vi "sensor integration for debug async v5.vi"() -> ()   [LabVIEW 2021]
uses:
  <vilib>/Analysis/NI_AALBase.lvlib
  65c7c016-c5e7-4ca0-8b30-908e1d77d521.vi
  <vilib>/Instr/_visa.llb/VISA Configure Serial Port (Instr).vi
  <vilib>/Analysis/baseanly.llb/Mean (DBL).vi
  controls/sensirion_flow_sensor_data.ctl
  type-defs/sensirion_data_with_time.ctl
  <extravilib>/ChannelInstances/Stream-t'sensirion_data_with_time.ctl'.lvlib
panel:
  out "sensor data timestamp":dbl
  out "logfile size (in MB)":dbl format="%.2f"
  out "sensirion data string":string
  in  "error in (no error)":errorcluster
  out "retry count":i32
  in  "read byte count (512)":u32=512
  in  "baud rate (576000)":u32=576000
  out "last loop time, ms":dbl
  out "mean refresh rate, Hz, n=250":dbl(knob) scale=0.05..100.0
  in  "loop delay, ms (0)":u32
  in  "expected num sensors (12)":i32=12
  out "sensor data array 7 - 12":T1[](array[typedef])=[{"flow rate \n(mL/min)"=0.0, "flow val. status"=FALSE, "temp.\n(C)"=0.0, "temp. val status"=FALSE, "air in \nline?"=FALSE, "high \nflow?"=FALSE, "flag. val status"=FALSE}, {"flow rate \n(mL/min)"=0.0, "flow val. status"=FALSE, "temp.\n(C)"=0.0, "temp. val status"=FALSE, "air in \nline?"=FALSE, "high \nflow?"=FALSE, "flag. val status"=FALSE}, {"flow rate \n(mL/min)"=0.0, "flow val. status"=TRUE, "temp.\n(C)"=0.0, "temp. val status"=TRUE, "air in \nline?"=FALSE, "high \nflow?"=FALSE, "flag. val status"=TRUE}, {"flow rate \n(mL/min)"=0.0, "flow val. status"=TRUE, "temp.\n(C)"=0.0, "temp. val status"=TRUE, "air in \nline?"=FALSE, "high \nflow?"=FALSE, "flag. val status"=TRUE}, {"flow rate \n(mL/min)"=0.0, "flow val. status"=TRUE, "temp.\n(C)"=0.0, "temp. val status"=TRUE, "air in \nline?"=FALSE, "high \nflow?"=FALSE, "flag. val status"=TRUE}, {"flow rate \n(mL/min)"=0.0, "flow val. status"=TRUE, "temp.\n(C)"=0.0, "temp. val status"=TRUE, "air in \nline?"=FALSE, "high \nflow?"=FALSE, "flag. val status"=TRUE}, {"flow rate \n(mL/min)"=0.0, "flow val. status"=TRUE, "temp.\n(C)"=0.0, "temp. val status"=TRUE, "air in \nline?"=FALSE, "high \nflow?"=FALSE, "flag. val status"=TRUE}, {"flow rate \n(mL/min)"=0.0, "flow val. status"=TRUE, "temp.\n(C)"=0.0, "temp. val status"=TRUE, "air in \nline?"=FALSE, "high \nflow?"=FALSE, "flag. val status"=TRUE}, {"flow rate \n(mL/min)"=0.0, "flow val. status"=TRUE, "temp.\n(C)"=0.0, "temp. val status"=TRUE, "air in \nline?"=FALSE, "high \nflow?"=FALSE, "flag. val status"=TRUE}, {"flow rate \n(mL/min)"=0.0, "flow val. status"=TRUE, "temp.\n(C)"=0.0, "temp. val status"=TRUE, "air in \nline?"=FALSE, "high \nflow?"=FALSE, "flag. val status"=TRUE}, {"flow rate \n(mL/min)"=0.0, "flow val. status"=TRUE, "temp.\n(C)"=0.0, "temp. val status"=TRUE, "air in \nline?"=FALSE, "high \nflow?"=FALSE, "flag. val status"=TRUE}, {"flow rate \n(mL/min)"=0.0, "flow val. status"=TRUE, "temp.\n(C)"=0.0, "temp. val status"=TRUE, "air in \nline?"=FALSE, "high \nflow?"=FALSE, "flag. val status"=TRUE}] {"temp.\n(C)" scale=20.0..30.0 scale format="%#_3g"; "flow rate \n(mL/min)" scale=0.0..4.0}
  out "sensor data array 1 - 6":T1[](array[typedef])=[{"flow rate \n(mL/min)"=0.0, "flow val. status"=FALSE, "temp.\n(C)"=0.0, "temp. val status"=FALSE, "air in \nline?"=FALSE, "high \nflow?"=FALSE, "flag. val status"=FALSE}, {"flow rate \n(mL/min)"=0.0, "flow val. status"=FALSE, "temp.\n(C)"=0.0, "temp. val status"=FALSE, "air in \nline?"=FALSE, "high \nflow?"=FALSE, "flag. val status"=FALSE}, {"flow rate \n(mL/min)"=0.0, "flow val. status"=TRUE, "temp.\n(C)"=0.0, "temp. val status"=TRUE, "air in \nline?"=FALSE, "high \nflow?"=FALSE, "flag. val status"=TRUE}, {"flow rate \n(mL/min)"=0.0, "flow val. status"=TRUE, "temp.\n(C)"=0.0, "temp. val status"=TRUE, "air in \nline?"=FALSE, "high \nflow?"=FALSE, "flag. val status"=TRUE}, {"flow rate \n(mL/min)"=0.0, "flow val. status"=TRUE, "temp.\n(C)"=0.0, "temp. val status"=TRUE, "air in \nline?"=FALSE, "high \nflow?"=FALSE, "flag. val status"=TRUE}, {"flow rate \n(mL/min)"=0.0, "flow val. status"=TRUE, "temp.\n(C)"=0.0, "temp. val status"=TRUE, "air in \nline?"=FALSE, "high \nflow?"=FALSE, "flag. val status"=TRUE}, {"flow rate \n(mL/min)"=0.0, "flow val. status"=TRUE, "temp.\n(C)"=0.0, "temp. val status"=TRUE, "air in \nline?"=FALSE, "high \nflow?"=FALSE, "flag. val status"=TRUE}, {"flow rate \n(mL/min)"=0.0, "flow val. status"=TRUE, "temp.\n(C)"=0.0, "temp. val status"=TRUE, "air in \nline?"=FALSE, "high \nflow?"=FALSE, "flag. val status"=TRUE}, {"flow rate \n(mL/min)"=0.0, "flow val. status"=TRUE, "temp.\n(C)"=0.0, "temp. val status"=TRUE, "air in \nline?"=FALSE, "high \nflow?"=FALSE, "flag. val status"=TRUE}, {"flow rate \n(mL/min)"=0.0, "flow val. status"=TRUE, "temp.\n(C)"=0.0, "temp. val status"=TRUE, "air in \nline?"=FALSE, "high \nflow?"=FALSE, "flag. val status"=TRUE}, {"flow rate \n(mL/min)"=0.0, "flow val. status"=TRUE, "temp.\n(C)"=0.0, "temp. val status"=TRUE, "air in \nline?"=FALSE, "high \nflow?"=FALSE, "flag. val status"=TRUE}, {"flow rate \n(mL/min)"=0.0, "flow val. status"=TRUE, "temp.\n(C)"=0.0, "temp. val status"=TRUE, "air in \nline?"=FALSE, "high \nflow?"=FALSE, "flag. val status"=TRUE}] {"temp.\n(C)" scale=20.0..30.0 scale format="%#_3g"; "flow rate \n(mL/min)" scale=0.0..3.0}
  out "error out":errorcluster
  in  "stop program":bool
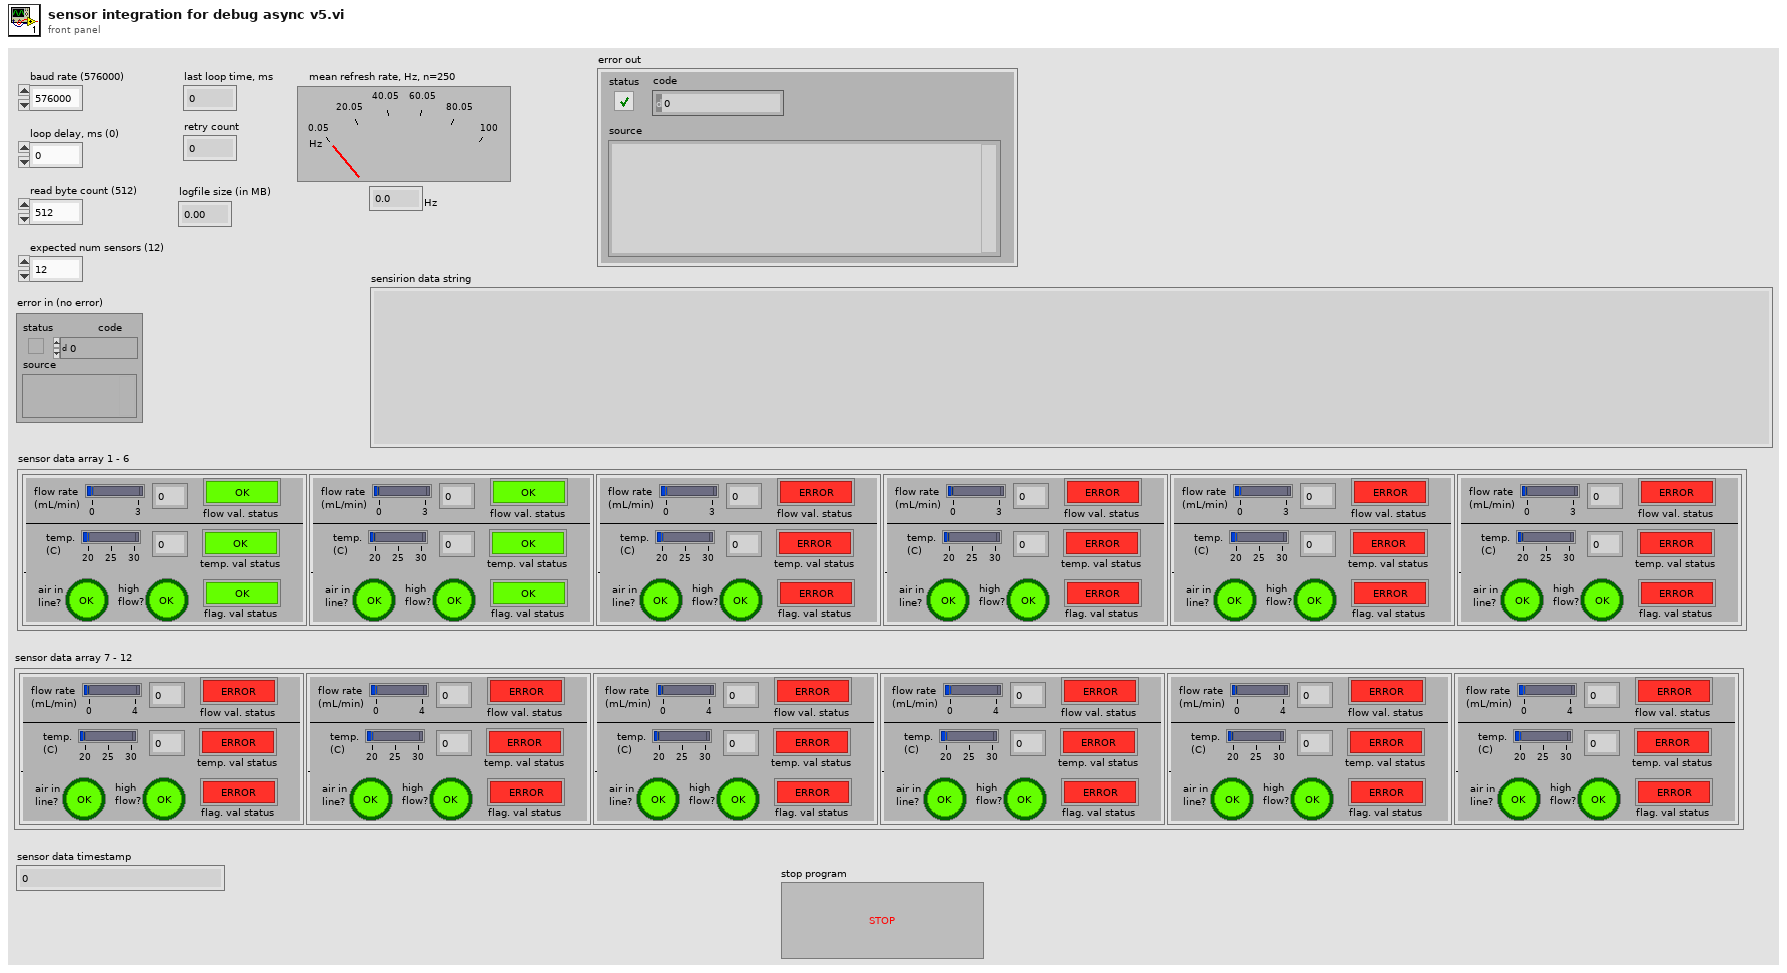
[diagram p1: front panel]
types:
  T1 = typedef "sensirion_flow_sensor_data.ctl" = cluster{"flow rate \n(mL/min)":dbl, "flow val. status":bool, "temp.\n(C)":dbl, "temp. val status":bool, "air in \nline?":bool, "high \nflow?":bool, "flag. val status":bool}
  T2 = enum16{"open", "replace", "create", "open or create", "replace or create", "replace or create with confirmation"}
  T3 = typedef "sensirion_data_with_time.ctl" = cluster{"sensor data array":T4[], "relative timestamp":dbl, "error":errorcluster}
  T4 = typedef "sensirion_flow_sensor_data.ctl" = cluster{"flow rate \n":dbl[unit], "flow val. status":bool, "temperature":dbl[unit], "temp. val status":bool, "air in line?":bool, "high flow?":bool, "flag. val status":bool}
  T5 = enum8{"Enabled", "Disabled", "Disabled and Grayed Out"}
  T6 = typedef "Stream-t'sensirion_data_with_time.ctl'.lvlib/)Channel.ctl" = refnum<queue>
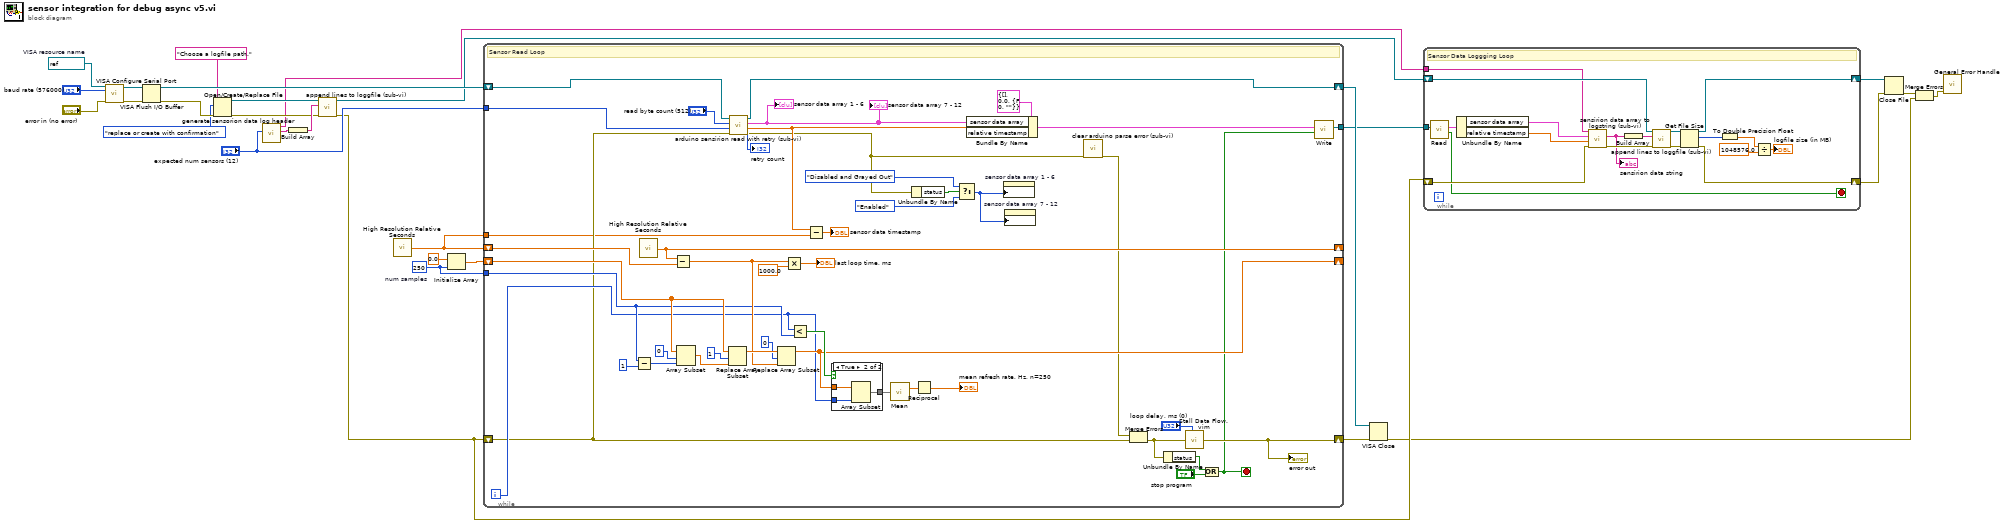
[diagram p0: block diagram]
diagram:
  w21 = 250  # num samples
  w28 = refnum<visa-resource-name> "COM3"  # VISA resource name
  n1 = call-poly "VISA Configure Serial Port"("VISA resource name"=w28, "baud rate (9600)"="baud rate (576000)", "error in (no error)"="error in (no error)") -> ("VISA resource name out"=w27:refnum<visa-resource-name>, "error out"=w26:errorcluster)  [unwired: 11 in]
  n2 = VISA Flush I/O Buffer(VISA resource name=w27, error in (no error)=w26) -> (VISA resource name out=w24:refnum<visa-resource-name>, error out=w25:errorcluster)  [unwired: 1 in]
  n3 = Open/Create/Replace File(error in=w25, prompt="Choose a logfile path.", operation (0:open)=T2."replace or create with confirmation") -> (refnum out=w15:refnum<file>, error out=w14:errorcluster)  [unwired: 3 in, 1 out]
  n4 = call "generate sensorion data log header.vi"("num sensors"="expected num sensors (12)") -> ("sensor data header string"=w17:string, "value format"=w1:string)  [unwired: 8 in, 1 out]
  n5 = Build Array(w17) -> (w16:string[])
  n6 = call "append lines to loggfile (sub-vi).vi"("error in (no error)"=w14, "string array"=w16, "file refnum"=w15) -> ("error out"=w10:errorcluster, "file refnum out"=w12:refnum<file>)  [unwired: 7 in]
  n7 = call <vilib>:"High Resolution Relative Seconds.vi"() -> ("relative seconds"=w4:dbl)
  n8 = Initialize Array(0.0 ("element"), w21) -> (w22:dbl[])
  n9 = while {
    shift-right: [w73] -> _
    shift-left: w4 -> [w72]
    shift-right: [w60] -> _
    shift-left: w22 -> [w68]
    shift-right: [w35] -> w9
    shift-left: w10 -> [w46]
    tunnel: w21 -> [w62]
    tunnel: "expected num sensors (12)" -> [w43]
    shift-right: [w30] -> w8
    shift-left: w24 -> [w31]
    tunnel: w4 -> [w40]
    tunnel: [w33] -> w3
    i -> [w59]
    stop <- w32 stop-if-true
    # "Sensor Read Loop"
    n10 = Subtract(x=w62, y=1) -> (x-y=w66:i32)
    n11 = call <vilib>:"High Resolution Relative Seconds.vi"() -> ("relative seconds"=w73:dbl)
    n12 = Subtract(x=w73, y=w72) -> (x-y=w64:dbl)
    n13 = Array Subset(array=w68, index=0, length=w66) -> (w71:dbl[])
    n14 = Replace Array Subset(array=w68, new element=w71, index=1) -> (w65:dbl[])
    n15 = call "arduino sensirion read with retry (sub-vi).vi"("error in (no error)"=w46, "expected num sensors (12)"=w43, "read byte count (512)"="read byte count (512)", "VISA resource name"=w31) -> ("error out"=w37:errorcluster, "relative timestamp"=w38:dbl, "sensor data array"=w39:T4[], "VISA resource name out"=w30:refnum<visa-resource-name>, "retry count"=→"retry count":i32)  [unwired: 3 in]
    "sensor data array 1 - 6" <- w39
    "sensor data array 7 - 12" <- w39
    n16 = Replace Array Subset(array=w65, new element=w64, index=0) -> (w60:dbl[])
    n17 = Multiply(x=w64, y=1000.0) -> (x*y=→"last loop time, ms":dbl)
    n18 = Less?(x=w59, y=w62) -> (x < y?=w61:bool)
    n19 = Subtract(x=w38, y=w40) -> (x-y=→"sensor data timestamp":dbl)
    n20 = case shown="True" w61 {
      tunnel: w60 -> [w75 w78]
      tunnel: w59 -> [_ w77]
      tunnel: [w75 w76] -> w58
      frame False {
      }
      frame True {
        n21 = Array Subset(array=w78, length=w77) -> (w76:dbl[])  [unwired: 1 in]
      }
    }
    n22 = call-poly <vilib>:"Mean.vi"("X"=w58) -> ("mean"=w57:dbl)  [unwired: 1 out]
    n23 = Unbundle By Name(w37) -> ("status"=w56:bool)
    n24 = Reciprocal(x=w57) -> (1/x=→"mean refresh rate, Hz, n=250":dbl)
    n25 = Select(t=T5."Disabled and Grayed Out" ("Disabled"), s=w56, f=T5."Enabled" ("Disabled")) -> (s? t:f=w54:T5)
    n26 = Bundle By Name(cluster=T3 {"sensor data array"=[], "relative timestamp"=0.0, "error"={"status"=FALSE, "code"=0, "source"=""}} ("Cluster"), "sensor data array"=w39, "relative timestamp"=w38) -> (w34:T3)
    n27 = property on="sensor data array 1 - 6" class="Arr (strict)"("DisabledEnum"=w54) -> ()  [unwired: 2 in, 2 out]
    n28 = property on="sensor data array 7 - 12" class="Arr (strict)"("DisabledEnum"=w54) -> ()  [unwired: 2 in, 2 out]
    n29 = call "clear arduino parse error (sub-vi).vi"("error in"=w37) -> ("error out"=w42:errorcluster)  [unwired: 10 in]
    n30 = Merge Errors(w42, w46) -> (w44:errorcluster)
    n31 = Unbundle By Name(w44) -> ("status"=w52:bool)
    n32 = call "Stall Data Flow.vim"("value in"=w44, "milliseconds to wait"="loop delay, ms (0)") -> ("value out"=w35:errorcluster)  [unwired: 1 out]
    "error out" <- w35
    n33 = Or(x=w52, y="stop program") -> (x .or. y?=w32:bool)
    n34 = call <extravilib>:"Write.vi"("last element? (F)"=w32, "element"=w34) -> ("channel"=w33:T6)  [unwired: 7 in, 2 out]
  }
  n35 = VISA Close(VISA resource name=w8, error in (no error)=w9) -> (error out=w7:errorcluster)
  n36 = while {
    shift-right: [w89] -> w2
    shift-left: w10 -> [w87]
    tunnel: w3 -> [w88]
    shift-right: [w90] -> w11
    shift-left: w12 -> [w91]
    tunnel: w1 -> [w79]
    stop <- w80 stop-if-true
    # "Sensor Data Loggging Loop"
    n37 = call <extravilib>:"Read.vi"("channel"=w88) -> ("last element?"=w80:bool, "element"=w85:T3)  [unwired: 6 in, 3 out]
    n38 = Unbundle By Name(w85) -> ("sensor data array"=w84:T4[], "relative timestamp"=w83:dbl)
    n39 = call "sensirion data array to logstring (sub-vi).vi"("error in"=w87, "timestamp in relative seconds"=w83, "sensor data array"=w84, "value format (%15s)"=w79) -> ("error out"=w86:errorcluster, "string out"=w81:string)  [unwired: 6 in]
    "sensirion data string" <- w81
    n40 = Build Array(w81) -> (w82:string[])
    n41 = call "append lines to loggfile (sub-vi).vi"("error in (no error)"=w86, "string array"=w82, "file refnum"=w91) -> ("error out"=w92:errorcluster, "file refnum out"=w97:refnum<file>)  [unwired: 7 in]
    n42 = Get File Size(file=w97, error in=w92) -> (refnum out=w90:refnum<file>, size (in bytes)=w96:i64, 0:w89:errorcluster)
    n43 = To Double Precision Float(number=w96) -> (double precision float=w95:dbl)
    n44 = Divide(x=w95, y=1048576.0) -> (x/y=→"logfile size (in MB)":dbl)
  }
  n45 = Close File(refnum=w11, error in=w2) -> (error out=w5:errorcluster)  [unwired: 1 out]
  n46 = Merge Errors(w5, w7) -> (w6:errorcluster)
  n47 = call <vilib>:"General Error Handler.vi"("error in (no error)"=w6) -> ()  [unwired: 10 in, 5 out]
